vi "Write Subpanel Refnum.vi"(7 "Force Overwrite? (F)":bool, 8 "error in (no error)":errorcluster, 10 "Protected Subpanel":T1, 11 "IViewModel In":refnum<class "IViewModel.lvclass">) -> (0 "error out":errorcluster, 3 "IViewModel Out":refnum<class "IViewModel.lvclass">)   [LabVIEW 2018, in "MVA Framework.lvlib" / "IViewModel.lvlib" / "IViewModel.lvclass"]
doc: "写入子面板引用"
uses:
  IViewModel.lvclass
  IViewable/ProtectedSubpanel/ProtectedSubpanel.lvclass
  IViewable/ProtectedSubpanel/Protected Subpanel Reference.ctl
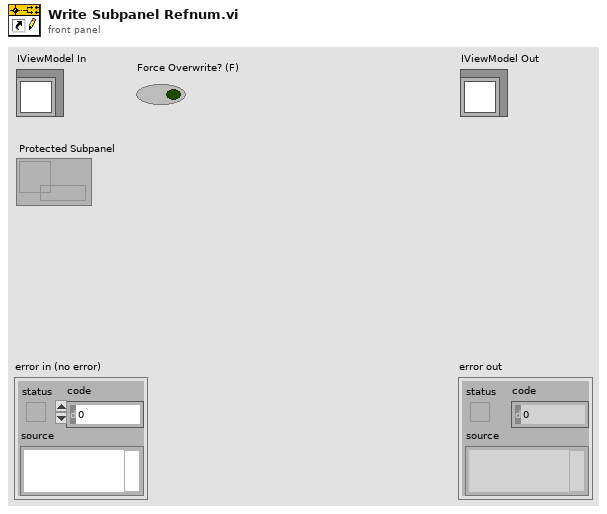
[diagram p1: front panel]
types:
  T1 = typedef "MVA Framework.lvlib/IViewable.lvlib/ProtectedSubpanel.lvclass/Protected Subpanel Reference.ctl" = refnum<data-value>
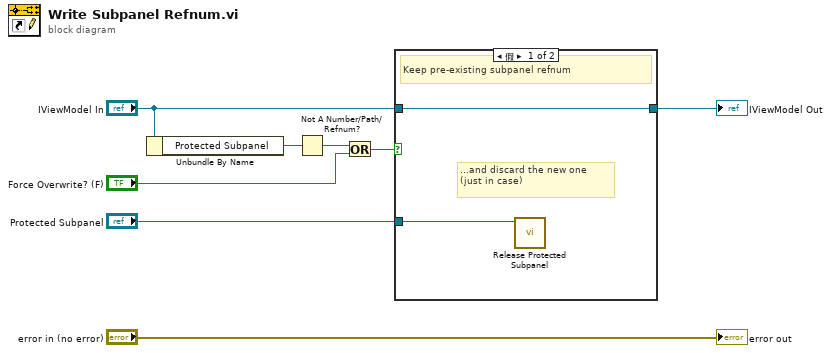
[diagram p0: block diagram]
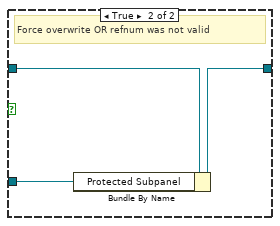
[diagram p2: hidden frame]
diagram:
  n1 = Unbundle By Name("IViewModel In") -> ("Protected Subpanel"=w5:T1)
  n2 = Not A Number/Path/Refnum?(number/path/refnum=w5) -> (NaN/Path/Refnum?=w4:bool)
  n3 = Or(x=w4, y="Force Overwrite? (F)") -> (x .or. y?=w1:bool)
  n4 = case shown="假" w1 {
    tunnel: [w10 w13] -> w7
    tunnel: "Protected Subpanel" -> [w9 w11]
    tunnel: "IViewModel In" -> [w10 w12]
    frame False {
      # "...and discard the new one\n(just in case)"
      # "Keep pre-existing subpanel refnum"
      n5 = call "Release Protected Subpanel.vi"("Protected Subpanel"=w9) -> ()  [unwired: 10 in, 1 out]
    }
    frame True {
      # "Force overwrite OR refnum was not valid"
      n6 = Bundle By Name(cluster=w12, "Protected Subpanel"=w11) -> (w13:refnum<class "IViewModel.lvclass">)
    }
  }
  "IViewModel Out" <- w7
  "error out" <- "error in (no error)"
